vi "SSL Referee to GUI Referee.vi"(11 "SSL Game Status":T1) -> (3 "GUI Game Status":T3 {"Time" format="%<%.3X %x>T"; "Blue Timeout Remaining" format="%<%M:%S>t"; "Yellow Timeout Remaining" format="%<%M:%S>t"; "Time Left" format="%<%M:%S>t"})   [LabVIEW 2023]
uses:
  SSL Referee Game Status.ctl
  Controls/SSL Referee.ctl
  SSL Referee Team Info.ctl
panel:
  # "Score"
  # "Red Cards"
  # "Yellow Cards"
  # "Timeouts Left"
  # "Timeout Remaining"
  # "Goalie ID"
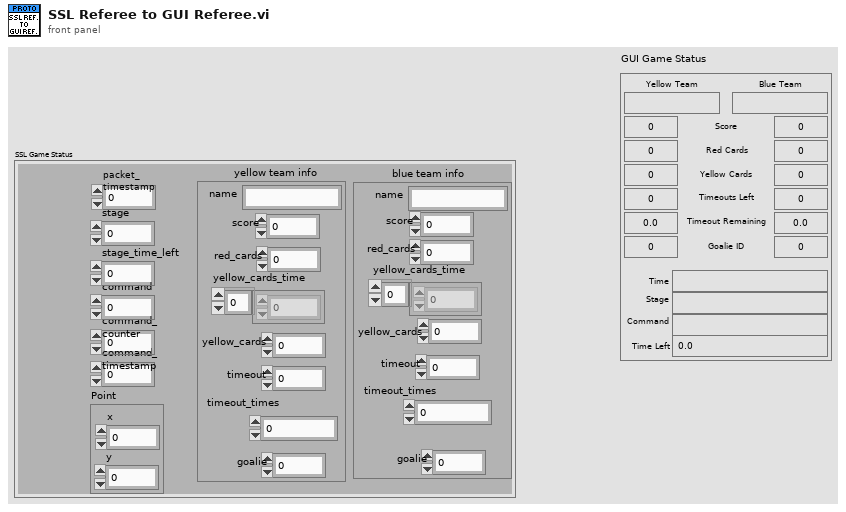
[diagram p1: front panel]
types:
  T1 = typedef "SSL Referee.ctl" = cluster{"packet_\ntimestamp":u64, "stage":u64, "stage_time_left":i32, "command ":u64, "command_\ncounter ":u32, "command_\ntimestamp":u64, "yellow team info":T2, "blue team info":T2, "Point":cluster{"x":sgl, "y":sgl}}
  T2 = typedef "SSL Referee Team Info.ctl" = cluster{"name":string, "score":u32, "red_cards":u32, "yellow_cards_time":u32[], "yellow_cards":u32, "timeout":u32, "timeout_times":u32, "goalie":u32}
  T3 = typedef "SSL Referee Game Status.ctl" = cluster{"Stage":string, "Command":string, "Time Left":dbl, "Yellow Team":string, "Blue Team":string, "Yellow Score":u32, "Blue Score":u32, "Yellow Red Cards":u32, "Blue Red Cards":u32, "Yellow Yellow Cards":u32, "Blue Yellow Cards":u32, "Yellow Timeouts Left":u32, "Blue Timeouts Left":u32, "Yellow Timeout Remaining":dbl, "Blue Timeout Remaining":dbl, "Yellow Goalie Id":u32, "Blue Goalie Id":u32, "Time":timestamp}
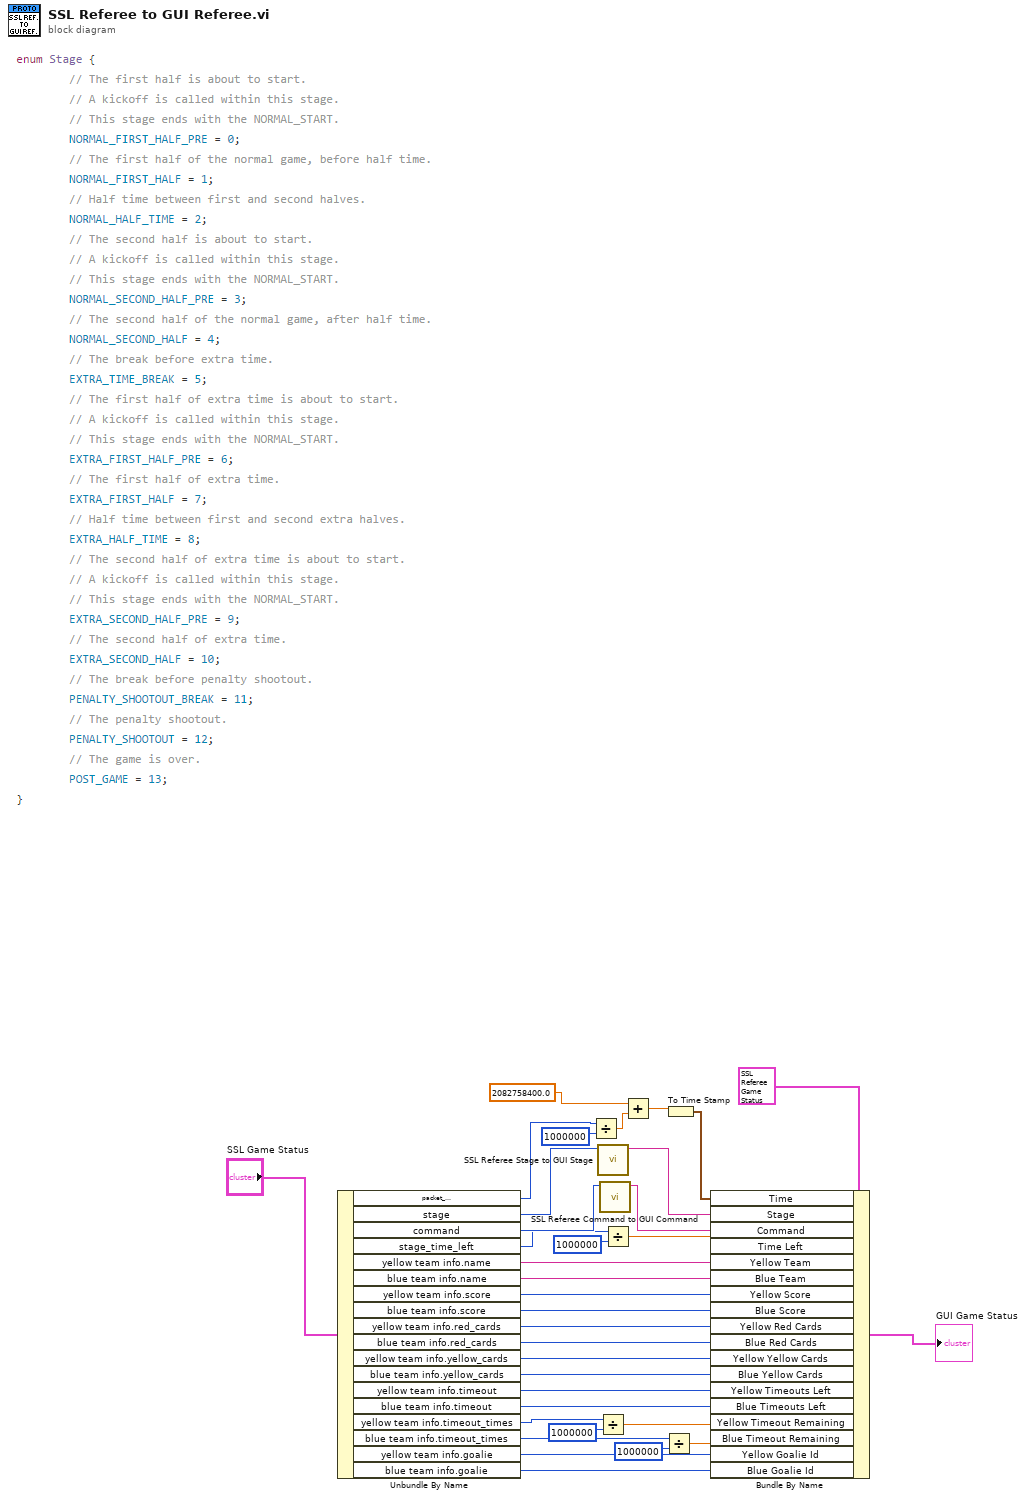
[diagram p0: block diagram]
diagram:
  n1 = Unbundle By Name("SSL Game Status") -> ("packet_\ntimestamp"=w3:u64, "stage"=w30:u64, "command"=w28:u64, "stage_time_left"=w26:i32, "yellow team info.name"=w1:string, "blue team info.name"=w34:string, "yellow team info.score"=w23:u32, "blue team info.score"=w22:u32, "yellow team info.red_cards"=w21:u32, "blue team info.red_cards"=w20:u32, "yellow team info.yellow_cards"=w19:u32, "blue team info.yellow_cards"=w18:u32, "yellow team info.timeout"=w17:u32, "blue team info.timeout"=w16:u32, "yellow team info.timeout_times"=w12:u32, "blue team info.timeout_times"=w8:u32, "yellow team info.goalie"=w15:u32, "blue team info.goalie"=w14:u32)
  n2 = Divide(x=w3, y=1000000) -> (x/y=w2:dbl)
  n3 = call "SSL Referee Stage to GUI Stage.vi"("stage"=w30) -> ("String"=w29:string)  [unwired: 10 in]
  n4 = Divide(x=w12, y=1000000) -> (x/y=w11:dbl)
  n5 = call "SSL Referee Command to GUI Command.vi"("stage"=w28) -> ("String"=w27:string)  [unwired: 10 in]
  n6 = Divide(x=w26, y=1000000) -> (x/y=w24:dbl)
  n7 = Add(x=2082758400.0, y=w2) -> (x+y=w6:dbl)
  n8 = Divide(x=w8, y=1000000) -> (x/y=w9:dbl)
  n9 = To Time Stamp(1:w6) -> (0:w5:timestamp)
  n10 = Bundle By Name(cluster=T3 {"Stage"="", "Command"="", "Time Left"=0.0, "Yellow Team"="", "Blue Team"="", "Yellow Score"=0, "Blue Score"=0, "Yellow Red Cards"=0, "Blue Red Cards"=0, "Yellow Yellow Cards"=0, "Blue Yellow Cards"=0, "Yellow Timeouts Left"=0, "Blue Timeouts Left"=0, "Yellow Timeout Remaining"=0.0, "Blue Timeout Remaining"=0.0, "Yellow Goalie Id"=0, "Blue Goalie Id"=0, "Time"=timestamp(0 s since 1904-01-01)} ("Game Status"), "Time"=w5, "Stage"=w29, "Command"=w27, "Time Left"=w24, "Yellow Team"=w1, "Blue Team"=w34, "Yellow Score"=w23, "Blue Score"=w22, "Yellow Red Cards"=w21, "Blue Red Cards"=w20, "Yellow Yellow Cards"=w19, "Blue Yellow Cards"=w18, "Yellow Timeouts Left"=w17, "Blue Timeouts Left"=w16, "Yellow Timeout Remaining"=w11, "Blue Timeout Remaining"=w9, "Yellow Goalie Id"=w15, "Blue Goalie Id"=w14) -> (→"GUI Game Status":T3)
